vi "Table, Delete Row Headers.vi"(7 "Enable (T)":bool=TRUE, 8 "error in":errorcluster, 11 "Tbl Refnum":refnum<vi>) -> (0 "error out":errorcluster, 3 "Tbl Refnum dup":refnum<vi>)   [LabVIEW 2010]
doc: "Shows all table rows plus an empty row.\nSince all rows are displayed, the vertical scrollbar is hidden."
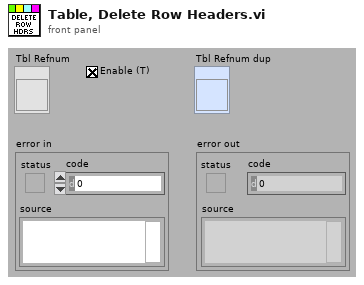
[diagram p1: front panel]
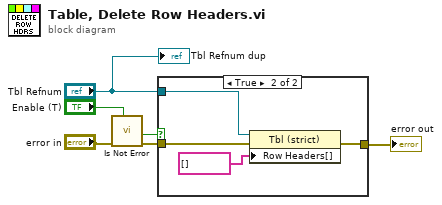
[diagram p0: block diagram]
diagram:
  n1 = call "Is Not Error.vi"("enable (T)"="Enable (T)", "error in"="error in") -> ("error out"=w3:errorcluster, "ready"=w4:bool)  [unwired: 4 in, 1 out]
  n2 = case shown="True" w4 {
    tunnel: [w7 w10] -> w6
    tunnel: "Tbl Refnum" -> [_ w11]
    tunnel: w3 -> [w7 w8]
    frame False {
    }
    frame True {
      n3 = property class="Tbl (strict)"(reference=w11, error in=w8, "Row Headers[]"=string[] [] ("Row Header Strings[]")) -> (error out=w10:errorcluster)  [unwired: 1 out]
    }
  }
  "error out" <- w6
  "Tbl Refnum dup" <- "Tbl Refnum"
